vi "Table-Find changed element.vi"(8 "error in (no error)":errorcluster, 10 "Table 2":string[][](array[string]), 11 "Table 1":string[][](array[string])) -> (0 "error out":errorcluster, 3 "Index of change":T1)   [LabVIEW 2020]
uses:
  <vilib>/Utility/miscctls.llb/LVRowAndColumnTypeDef.ctl
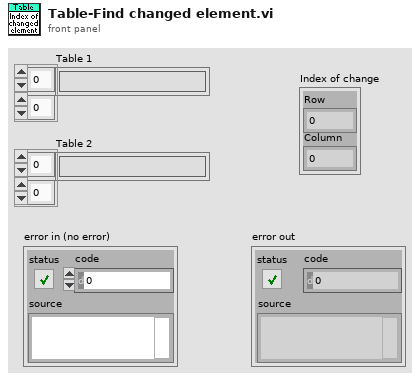
[diagram p1: front panel]
types:
  T1 = typedef "LVRowAndColumnTypeDef.ctl" = cluster{"Row":i32, "Column":i32}
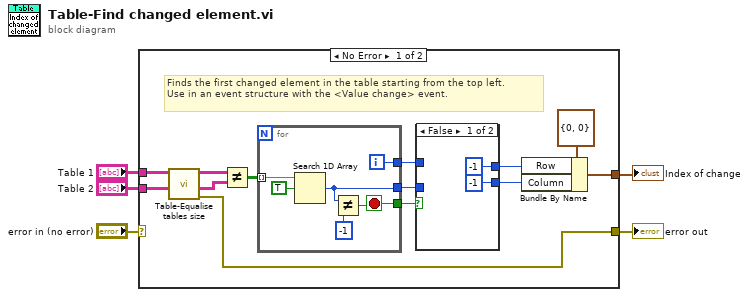
[diagram p0: block diagram]
diagram:
  n1 = case shown="No Error" "error in (no error)" {
    selector: "error in (no error)" -> [_ w29]
    tunnel: [w12 _] -> w5
    tunnel: "Table 1" -> [w10 _]
    tunnel: "Table 2" -> [w8 _]
    tunnel: [w6 w29] -> w1
    frame No Error {
      # "Finds the first changed element in the table starting from the top left.\nUse in an event structure with the <Value change> event."
      n2 = call "Table-Equalise tables size.vi"("Tabe 2 (in)"=w8, "Table 1 (in)"=w10) -> ("error out"=w6:errorcluster, "Tabe 2"=w7:string[][], "Table 1"=w9:string[][])  [unwired: 7 in]
      n3 = Not Equal?(x=w9, y=w7) -> (x != y?=w15:bool[][])
      n4 = for {
        tunnel: w15 -> [w28] mode=indexing
        tunnel: [w25] -> w18
        tunnel: [w26] -> w17
        tunnel: [w23] -> w16
        i -> [w26]
        stop <- w23 stop-if-true
        n5 = Search 1D Array(1D array=w28, element=TRUE) -> (index of element=w25:i32)  [unwired: 1 in]
        n6 = Not Equal?(x=w25, y=-1) -> (x != y?=w23:bool)
      }
      n7 = case shown="False" w16 {
        tunnel: w17 -> [_ w22]
        tunnel: w18 -> [_ w21]
        tunnel: [-1 w22] -> w13
        tunnel: [-1 ("index of element") w21] -> w11
        frame False {
        }
        frame True {
        }
      }
      n8 = Bundle By Name(cluster=T1 {"Row"=0, "Column"=0} ("Selection Start"), "Row"=w13, "Column"=w11) -> (w12:T1)
    }
    frame Error {
    }
  }
  "Index of change" <- w5
  "error out" <- w1
